vi "Read Configuration.vi"(8 "error in (no error)":errorcluster, 11 "ADAS PE Template Controller in":refnum<class "PE Controller.lvclass">) -> (0 "error out":errorcluster, 2 "Configuration":T1, 3 "ADAS PE Template Controller out":refnum<class "PE Controller.lvclass">)   [LabVIEW 2020, in "ADAS PE Template.lvlib" / "PE Controller.lvclass"]
doc: "<b>Read Configuration</b>\nThis method directly returns the <b>Configuration.ct</b> stored in the class data of this plugin's controller."
uses:
  PE Controller.lvclass
  PE/Configuration.ctl
  PE Controller.lvclass/PE Controller.ctl
  PE/ADAS PE Template.lvclass
panel:
  # "#via_ignore"
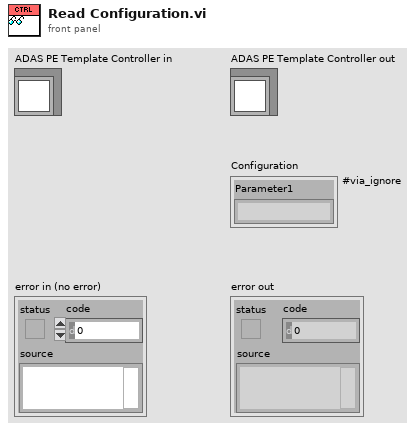
[diagram p1: front panel]
types:
  T1 = typedef "ADAS PE Template.lvlib/ADAS PE Template.lvclass/Configuration.ctl" = cluster{"Parameter1":string}
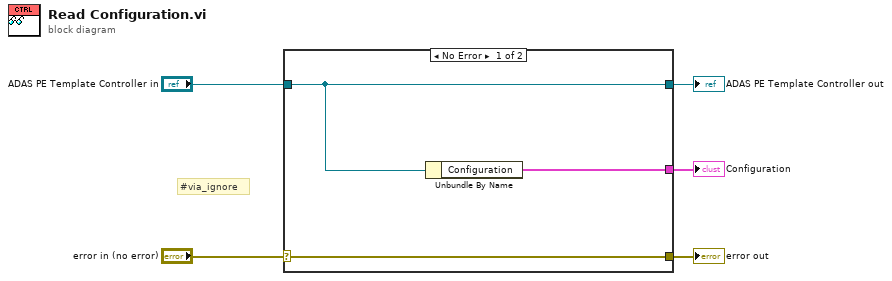
[diagram p0: block diagram]
diagram:
  # "#via_ignore"
  n1 = case shown="No Error" "error in (no error)" {
    selector: "error in (no error)" -> [w8 w9]
    tunnel: [w8 w9] -> w4
    tunnel: [w6 w10] -> w2
    tunnel: "ADAS PE Template Controller in" -> [w6 w10]
    tunnel: [w7 _] -> w1
    frame No Error {
      n2 = Unbundle By Name(w6) -> ("Configuration"=w7:T1)
    }
    frame Error {
    }
  }
  "error out" <- w4
  "ADAS PE Template Controller out" <- w2
  "Configuration" <- w1
